vi "DistancesData.vi"(11 "Distances":T2(array[cluster])) -> (3 "Distances 2":T2(array[cluster]))   [LabVIEW 2013]
uses:
  Program Files (x86)/National Instruments/LabVIEW 2013/examples/FRC/Vision/2014 Target Detection/TargetType.ctl
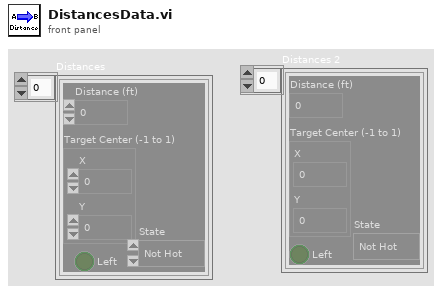
[diagram p1: front panel]
types:
  T1 = typedef "TargetType.ctl" = enum16{"Not Hot", "Hot"}
  T2 = cluster{"Distance (ft)":dbl, "Target Center (-1 to 1)":cluster{"X":dbl, "Y":dbl}, "Left":bool, "State":T1}[]
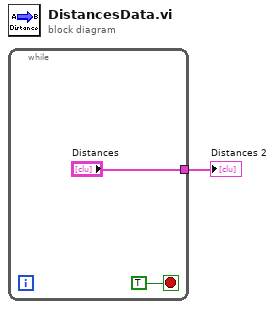
[diagram p0: block diagram]
diagram:
  n1 = while {
    tunnel: ["Distances"] -> w1
    stop <- TRUE stop-if-true
  }
  "Distances 2" <- w1
